vi "读取文本文件.vi"() -> ()   [LabVIEW 2010]
panel:
  in  "计数":i32
  out "文本":string
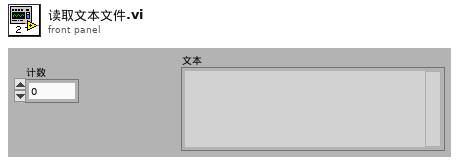
[diagram p1: front panel]
types:
  T1 = enum16{"open", "replace", "create", "open or create", "replace or create", "replace or create with confirmation"}
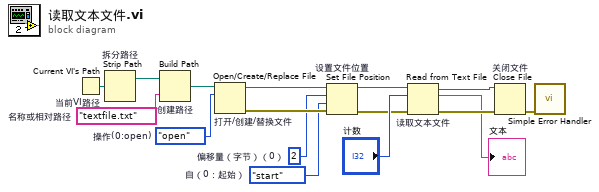
[diagram p0: block diagram]
diagram:
  w1 = "textfile.txt"  # 名称或相对路径
  w2 = enum16{"start", "end", "current"}."start"  # 自（0：起始）
  w3 = i64 2  # 偏移量（字节）（0）
  w10 = T1."open"  # 操作(0:open)
  n1 = Current VI's Path "当前VI路径"() -> (path=w16:path)
  n2 = Strip Path "拆分路径"(path=w16) -> (stripped path=w11:path)  [unwired: 1 out]
  n3 = Build Path "创建路径"(base path=w11, name or relative path=w1) -> (appended path=w15:path)
  n4 = Open/Create/Replace File "打开/创建/替换文件"(file path (use dialog)=w15, operation (0:open)=w10) -> (refnum out=w4:refnum<file>, error out=w7:errorcluster)  [unwired: 4 in, 1 out]
  n5 = Set File Position "设置文件位置"(offset (in bytes) (0)=w3, refnum=w4, from (0:start)=w2, error in=w7) -> (refnum out=w5:refnum<file>, error out=w6:errorcluster)
  n6 = Read from Text File "读取文本文件"(file (use dialog)=w5, count="计数", error in=w6) -> (refnum out=w14:refnum<file>, text=→"文本":string, error out=w13:errorcluster)  [unwired: 1 in, 1 out]
  n7 = Close File "关闭文件"(refnum=w14, error in=w13) -> (error out=w12:errorcluster)  [unwired: 1 out]
  n8 = call <vilib>:"Simple Error Handler.vi"("error in (no error)"=w12) -> ()  [unwired: 4 in, 5 out]
